vi "readparams2.vi"(0 "Port In":refnum<visa-resource-name>="ASRL18::INSTR", 3 "var query":string="frETWIUdmxlust[]^knXcwFqAPORj*<>,/b;:UdmD", 7 "error in":errorcluster, 11 "Get F&A":bool, 12 "Prog Chan?":bool, 14 "ChSt":bool) -> (1 "RFonA":bool, 2 "RFonB":bool, 4 "LevA":bool, 5 "LevB":bool, 8 "FchA":dbl, 9 "FchB":dbl, 13 "ComError":bool, 16 "AdBm":dbl, 17 "BdBm":dbl, 20 "Port Out":refnum<visa-resource-name>="ASRL18::INSTR", 21 "NowLevel":bool, 23 "cluster":T1, 24 "NowFreq":dbl, 25 "NowdBm":dbl, 27 "error out":errorcluster)   [LabVIEW 2012]
uses:
  <vilib>/Utility/error.llb/DialogType.ctl
  <vilib>/Instr/_visa.llb/VISA Configure Serial Port (Instr).vi
panel:
  out "NowRFon":bool
  out "result":i32
  out "element":dbl
  out "Array":dbl[](array[numeric])
  out "output":string="C1f?a?C0"
  # "Ch 0(A)"
  # "Ch1(B)"
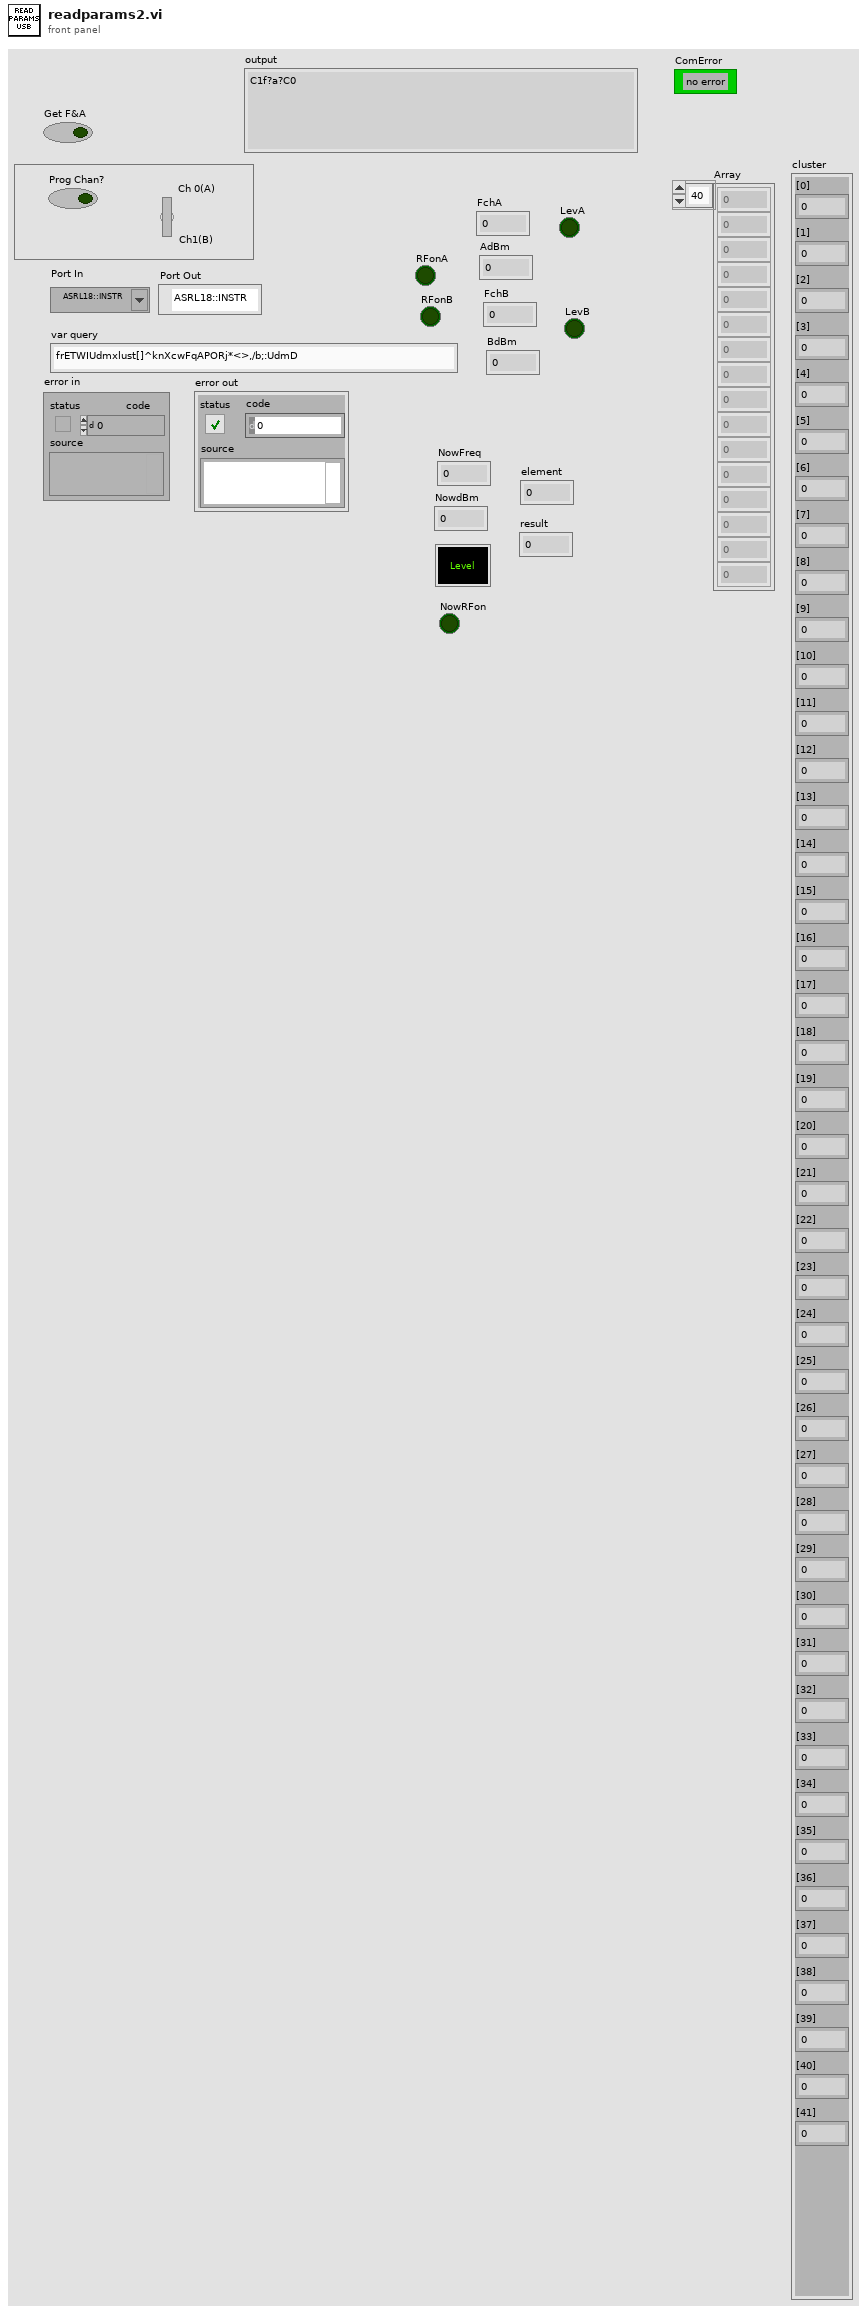
[diagram p1: front panel]
types:
  T1 = cluster{"[0]":dbl, "[1]":dbl, "[2]":dbl, "[3]":dbl, "[4]":dbl, "[5]":dbl, "[6]":dbl, "[7]":dbl, "[8]":dbl, "[9]":dbl, "[10]":dbl, "[11]":dbl, "[12]":dbl, "[13]":dbl, "[14]":dbl, "[15]":dbl, "[16]":dbl, "[17]":dbl, "[18]":dbl, "[19]":dbl, "[20]":dbl, "[21]":dbl, "[22]":dbl, "[23]":dbl, "[24]":dbl, "[25]":dbl, "[26]":dbl, "[27]":dbl, "[28]":dbl, "[29]":dbl, "[30]":dbl, "[31]":dbl, "[32]":dbl, "[33]":dbl, "[34]":dbl, "[35]":dbl, "[36]":dbl, "[37]":dbl, "[38]":dbl, "[39]":dbl, "[40]":dbl, "[41]":dbl}
  T2 = typedef "DialogType.ctl" = u16
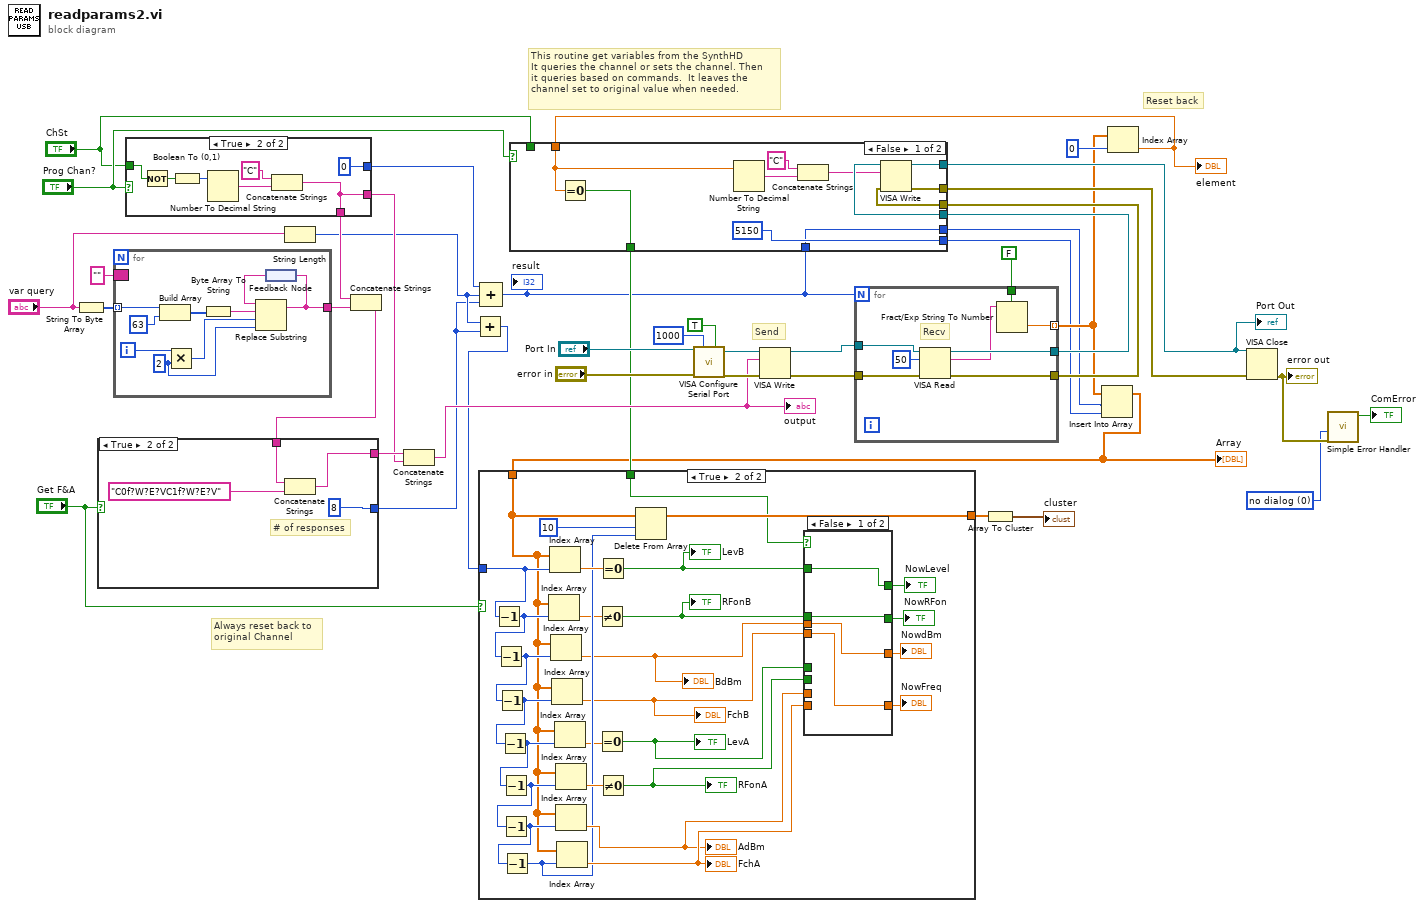
[diagram p0: block diagram]
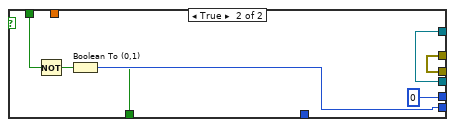
[diagram p2: hidden frame]
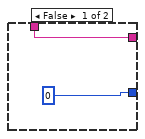
[diagram p5: hidden frame]
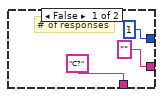
[diagram p6: hidden frame]
diagram:
  w2 = T2 0 items=["no dialog", "OK message", "continue or stop message", "OK message + warnings", "continue/stop + warnings"] ("type of dialog (OK msg:1)")
  # "This routine get variables from the SynthHD\nIt queries the channel or sets the channel. Then\nit queries based on commands.  It leaves the\nchannel set to original value when needed."
  # "Reset back"
  # "Always reset back to\noriginal Channel"
  # "Send"
  n1 = String To Byte Array(string="var query") -> (unsigned byte array=w33:u8[])
  n2 = for {
    tunnel: w33 -> [w51] mode=indexing
    tunnel: [w43] -> w31
    border: "" ("result string") -> [_]
    i -> [w47]
    w45 = 2 ("y")
    n3 = Build Array(w51, u8 63 ("element")) -> (w49:u8[])
    n4 = Multiply(x=w47, y=w45) -> (x*y=w46:i32)
    n5 = Byte Array To String(unsigned byte array=w49) -> (string=w48:string)
    n6 = feedback #1() -> (w44:string)
    n7 = Replace Substring(2:w45, 3:w46, 4:w48, 5:w44) -> (1:w43:string)  [unwired: 1 out]
    n8 = feedback-in #1(w43) -> ()
  }
  n9 = case shown="True" "Prog Chan?" {
    tunnel: ["C?" ("string") w56] -> w30
    tunnel: "ChSt" -> [_ w58]
    tunnel: ["" w56] -> w26
    tunnel: [1 ("y") 0 ("y")] -> w13
    frame False {
      # "# of responses"
    }
    frame True {
      n10 = Not(x=w58) -> (.not. x?=w57:bool)
      n11 = Boolean To (0,1)(Boolean=w57) -> (0, 1=w61:i16)
      n12 = Number To Decimal String(number=w61) -> (decimal integer string=w60:string)  [unwired: 1 in]
      n13 = Concatenate Strings("C" ("element"), w60) -> (w56:string)
    }
  }
  n14 = String Length(string="var query") -> (length=w7:i32)
  n15 = Concatenate Strings(w30, w31) -> (w29:string)
  n16 = case shown="True" "Get F&A" {
    tunnel: [w62 w64] -> w27
    tunnel: [0 ("y") 8 ("y")] -> w5
    tunnel: w29 -> [w62 w65]
    frame False {
    }
    frame True {
      # "# of responses"
      n17 = Concatenate Strings(w65, "C0f?W?E?VC1f?W?E?V" ("string")) -> (w64:string)
    }
  }
  n18 = Concatenate Strings(w27, w26) -> (w25:string)
  "output" <- w25
  n19 = Add(x=w7, y=w5) -> (x+y=w6:i32)
  n20 = Compound Arithmetic op=ADD(w13, w7, w5) -> (w8:i32)
  "result" <- w8
  n21 = call-poly "VISA Configure Serial Port"("VISA resource name"="Port In", "timeout (10sec)"=u32 1000, "Enable Termination\nChar (T)"=TRUE ("Enable Termination\nChar (T)"), "error in (no error)"="error in") -> ("VISA resource name out"=w38:refnum<visa-resource-name>, "error out"=w39:errorcluster)  [unwired: 5 in, 5 out]
  n22 = VISA Write(VISA resource name=w38, write buffer=w25, error in (no error)=w39) -> (VISA resource name out=w36:refnum<visa-resource-name>, error out=w37:errorcluster)  [unwired: 1 out]
  n23 = for {
    N: w8 -> [_]
    tunnel: w37 -> [w74]
    tunnel: w36 -> [w73]
    tunnel: [w72] -> w17
    tunnel: [w71] -> w19
    tunnel: [w69] -> w12 mode=indexing
    tunnel: FALSE ("use system decimal point (T)") -> [w68]
    # "Recv"
    n24 = VISA Read(VISA resource name=w73, byte count=u32 50, error in (no error)=w74) -> (VISA resource name out=w72:refnum<visa-resource-name>, read buffer=w70:string, error out=w71:errorcluster)  [unwired: 1 out]
    n25 = Fract/Exp String To Number(use system decimal point (T)=w68, string=w70) -> (number=w69:dbl)  [unwired: 2 in, 1 out]
  }
  n26 = Index Array(array=w12, index=0) -> (element=w14:dbl)
  "element" <- w14
  n27 = case shown="False" "Prog Chan?" {
    tunnel: "ChSt" -> [_ w87]
    tunnel: [w86 w87] -> w21
    tunnel: w14 -> [w83 _]
    tunnel: w17 -> [w82 w91]
    tunnel: w19 -> [w81 w92]
    tunnel: [w80 w92] -> w18
    tunnel: [w79 w91] -> w16
    tunnel: [w76 0 ("y")] -> w10
    tunnel: [5150 ("y") w89] -> w9
    tunnel: w8 -> [w76 _]
    frame False {
      n28 = Equal To 0?(x=w83) -> (x = 0?=w86:bool)
      n29 = Number To Decimal String(number=w83) -> (decimal integer string=w85:string)  [unwired: 1 in]
      n30 = Concatenate Strings("C" ("element"), w85) -> (w78:string)
      n31 = VISA Write(VISA resource name=w82, write buffer=w78, error in (no error)=w81) -> (VISA resource name out=w79:refnum<visa-resource-name>, error out=w80:errorcluster)  [unwired: 1 out]
    }
    frame True {
      n32 = Not(x=w87) -> (.not. x?=w88:bool)
      n33 = Boolean To (0,1)(Boolean=w88) -> (0, 1=w89:i16)
    }
  }
  "Port Out" <- w16
  n34 = Insert Into Array(array=w12, index=w10, new element=w9) -> (w11:dbl[])
  "Array" <- w11
  n35 = case shown="True" "Get F&A" {
    tunnel: w11 -> [w93 w107]
    tunnel: w6 -> [_ w117]
    tunnel: [w93 w119] -> w20
    tunnel: w21 -> [_ w113]
    frame False {
    }
    frame True {
      n36 = Decrement(x=w117) -> (x-1=w121:i32)
      n37 = Decrement(x=w121) -> (x-1=w120:i32)
      n38 = Decrement(x=w120) -> (x-1=w112:i32)
      n39 = Decrement(x=w112) -> (x-1=w111:i32)
      n40 = Decrement(x=w111) -> (x-1=w109:i32)
      n41 = Decrement(x=w109) -> (x-1=w108:i32)
      n42 = Decrement(x=w108) -> (x-1=w103:i32)
      n43 = Index Array(array=w107, index=w121) -> (element=w96:dbl)
      n44 = Index Array(array=w107, index=w117) -> (element=w110:dbl)
      n45 = Index Array(array=w107, index=w120) -> (element=w97:dbl)
      "BdBm" <- w97
      n46 = Index Array(array=w107, index=w112) -> (element=w98:dbl)
      "FchB" <- w98
      n47 = Index Array(array=w107, index=w111) -> (element=w102:dbl)
      n48 = Index Array(array=w107, index=w109) -> (element=w104:dbl)
      n49 = Index Array(array=w107, index=w108) -> (element=w105:dbl)
      "AdBm" <- w105
      n50 = Index Array(array=w107, index=w103) -> (element=w106:dbl)
      "FchA" <- w106
      n51 = Not Equal To 0?(x=w96) -> (x != 0?=w95:bool)
      "RFonB" <- w95
      n52 = Equal To 0?(x=w102) -> (x = 0?=w99:bool)
      "LevA" <- w99
      n53 = Equal To 0?(x=w110) -> (x = 0?=w94:bool)
      "LevB" <- w94
      n54 = Not Equal To 0?(x=w104) -> (x != 0?=w100:bool)
      "RFonA" <- w100
      n55 = Delete From Array(array=w107, length=10, index=w103) -> (array with subset deleted=w119:dbl[])  [unwired: 1 out]
      n56 = case shown="False" w113 {
        tunnel: [w124 w129] -> w115
        tunnel: [w125 w128] -> w116
        tunnel: [w122 w126] -> w114
        tunnel: w105 -> [_ w129]
        tunnel: w106 -> [_ w128]
        tunnel: [w123 w127] -> w101
        tunnel: w100 -> [_ w127]
        tunnel: w99 -> [_ w126]
        tunnel: w98 -> [w125 _]
        tunnel: w97 -> [w124 _]
        tunnel: w95 -> [w123 _]
        tunnel: w94 -> [w122 _]
        frame False {
        }
        frame True {
        }
      }
      "NowdBm" <- w115
      "NowFreq" <- w116
      "NowLevel" <- w114
      "NowRFon" <- w101
    }
  }
  n57 = Array To Cluster(array=w20) -> (cluster=→"cluster":T1)
  n58 = VISA Close(VISA resource name=w16, error in (no error)=w18) -> (error out=w3:errorcluster)
  "error out" <- w3
  n59 = call <vilib>:"Simple Error Handler.vi"("type of dialog (OK msg:1)"=w2, "error in (no error)"=w3) -> ("error?"=→"ComError":bool)  [unwired: 7 out]
